vi "Load_Digits.vi"(8 "error in":errorcluster caption="entrée d'erreur") -> (0 "error out":errorcluster caption="sortie d'erreur", 3 "String 3DArray":cluster{"Data":string[][]}[](array[cluster]))   [LabVIEW 2020]
doc: "Data Set Characteristics :\n\nNumber of Instances : 5620\n\nNumber of Attributes : 64\n\nAttribute Information : 8x8 image of integer pixels in the range 0..16.\n\nMissing Attribute Values : None\n\nCreator : Alpaydin (alpaydin ‘@’ boun.edu.tr)\n\nDate : July; 1998\n\nThis is a copy of the test set of the UCI ML hand-written digits datasets https://archive.ics.uci.edu/ml/datasets/Optical+Recognition+of+Handwritten+Digits\n\nThe data set contains images of hand-written digits: 10 classes where each class refers to a digit.\n\nPreprocessing programs made available by NIST were used to extract normalized bitmaps of handwritten digits from a preprinted form. From a total of 43 people, 30 contributed to the training set and different 13 to the test set. 32x32 bitmaps are divided into nonoverlapping blocks of 4x4 and the number of on pixels are counted in each block. This generates an input matrix of 8x8 where each element is an integer in the range 0..16. This reduces dimensionality and gives invariance to small distortions.\n\nFor info on NIST preprocessing routines, see M. D. Garris, J. L. Blue, G. T. Candela, D. L. Dimmick, J. Geist, P. J. Grother, S. A. Janet, and C. L. Wilson, NIST Form-Based Handprint Recognition System, NISTIR 5469, 1994."
uses:
  Load_Digits.lvclass
panel:
  out "Load_Digits en sortie":refnum<class "Load_Digits.lvclass">
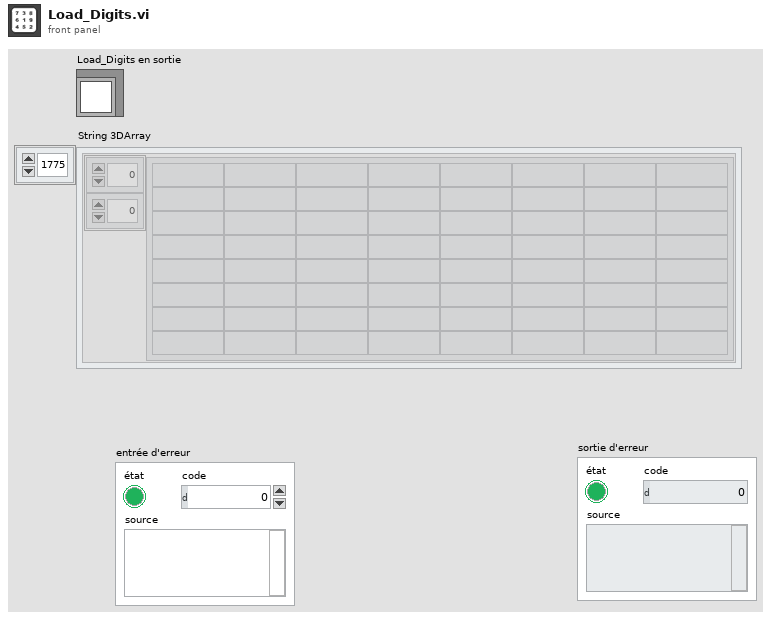
[diagram p1: front panel]
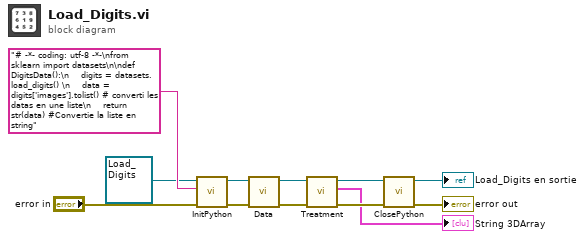
[diagram p0: block diagram]
diagram:
  n1 = call-dynamic "InitPython.vi"("error in (no error)"="error in", "Python Instruction"="# -*- coding: utf-8 -*-\nfrom sklearn import datasets\n\ndef DigitsData():\n    digits = datasets.load_digits() \n    data = digits['images'].tolist() # converti les datas en une liste\n    return str(data) #Convertie la liste en string", "Scikit-learn en entrée"=refnum<class "Load_Digits.lvclass"> refnum ("Load_Digits.lvclass")) -> ("error out"=w7:errorcluster, "Scikit-learn en sortie"=w8:refnum<class "Load_Digits.lvclass">)  [unwired: 7 in]
  n2 = call-dynamic "Data.vi"("error in (no error)"=w7, "Load_Digits en entrée"=w8) -> ("error out"=w5:errorcluster, "Load_Digits en sortie"=w6:refnum<class "Load_Digits.lvclass">)  [unwired: 8 in]
  n3 = call-dynamic "Treatment.vi"("error in (no error)"=w5, "Load_Digits en entrée"=w6) -> ("error out"=w3:errorcluster, "String 3DArray"=→"String 3DArray":cluster{"Data":string[][]}[], "Load_Digits en sortie"=w4:refnum<class "Load_Digits.lvclass">)  [unwired: 7 in]
  n4 = call-dynamic "ClosePython.vi"("error in (no error)"=w3, "Scikit-learn en entrée"=w4) -> ("error out"=→"error out":errorcluster, "Scikit-learn en sortie"=→"Load_Digits en sortie":refnum<class "Load_Digits.lvclass">)  [unwired: 8 in]
